vi "Read alarm XML.vi"(0 "map in":T2) -> (7 "map out":T1, 8 "data":T3, 9 "change?":bool)   [LabVIEW 2016, in "Alarm interface.lvlib"]
uses:
  Alarm interface.lvlib
panel:
  out "报警":T4
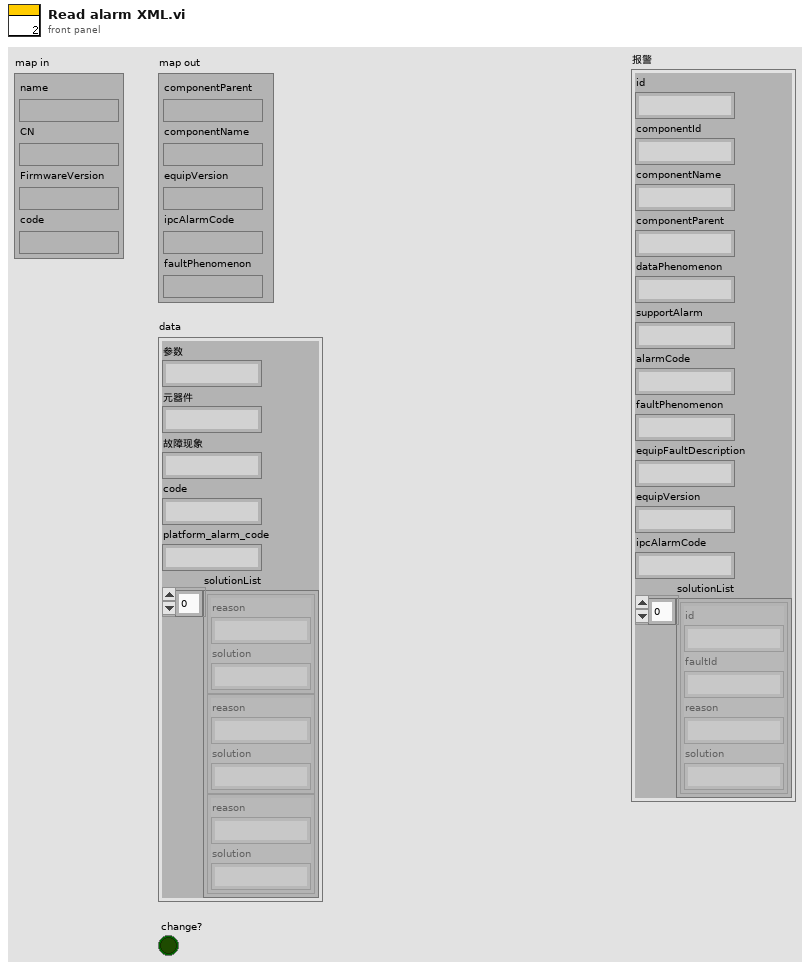
[diagram p1: front panel]
types:
  T1 = typedef "Alarm interface.lvlib/map out.ctl" = cluster{"componentParent":string, "componentName":string, "equipVersion":string, "ipcAlarmCode":string, "faultPhenomenon":string}
  T2 = typedef "Alarm interface.lvlib/map in.ctl" = cluster{"name":string, "CN":string, "FirmwareVersion":string, "code":string}
  T3 = typedef "Alarm interface.lvlib/报警短信语音交互.ctl" = cluster{"参数":string, "元器件":string, "故障现象":string, "code":string, "platform_alarm_code":string, "solutionList":cluster{"reason":string, "solution":string}[]}
  T4 = cluster{"id":string, "componentId":string, "componentName":string, "componentParent":string, "dataPhenomenon":string, "supportAlarm":string, "alarmCode":string, "faultPhenomenon":string, "equipFaultDescription":string, "equipVersion":string, "ipcAlarmCode":string, "solutionList":cluster{"id":string, "faultId":string, "reason":string, "solution":string}[]}
  T5 = cluster{"componentParent":string, "componentName":string, "equipVersion":string, "Code":string}
  T6 = cluster{"id":string, "componentId":string, "componentName":string, "componentParent":string, "dataPhenomenon":string, "supportAlarm":string, "alarmCode":string, "faultPhenomenon":string, "equipFaultDescription":string, "equipVersion":string, "ipcAlarmCode":string, "solutionList":cluster{"id":string, "faultId":string, "reason":string, "solution":string}[]}[]
  T7 = cluster{"id":string, "faultId":string, "reason":string, "solution":string}[]
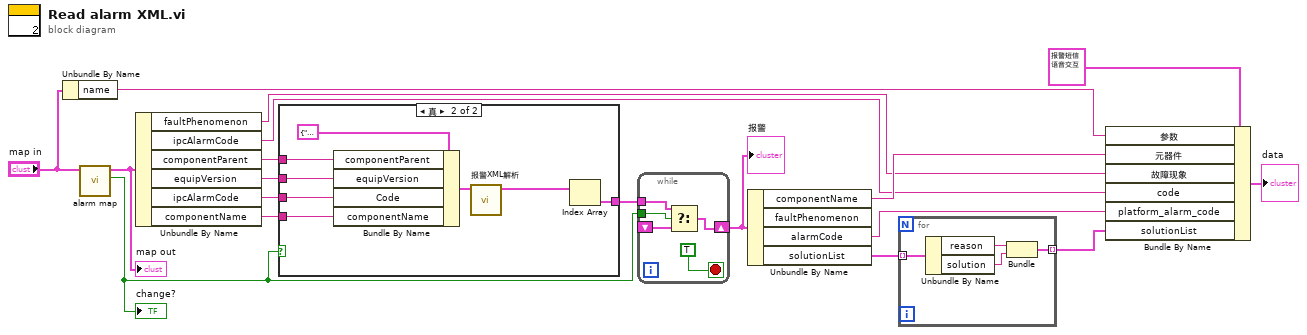
[diagram p0: block diagram]
diagram:
  n1 = Unbundle By Name("map in") -> ("name"=w4:string)
  n2 = call "alarm map.vi"("map in"="map in") -> ("change?"=w6:bool, "map out"=w7:T1)  [unwired: 8 in, 1 out]
  "map out" <- w7
  "change?" <- w6
  n3 = Unbundle By Name(w7) -> ("faultPhenomenon"=w3:string, "ipcAlarmCode"=w2:string, "componentParent"=w17:string, "equipVersion"=w18:string, "ipcAlarmCode"=w8:string, "componentName"=w1:string)
  n4 = case shown="真" w6 {
    tunnel: w17 -> [_ w26]
    tunnel: w18 -> [_ w25]
    tunnel: w8 -> [_ w24]
    tunnel: [_ w22] -> w15
    tunnel: w1 -> [_ w19]
    frame False {
    }
    frame True {
      n5 = Bundle By Name(cluster=T5 {"componentParent"="", "componentName"="", "equipVersion"="", "Code"=""} ("筛选输入"), "componentParent"=w26, "equipVersion"=w25, "Code"=w24, "componentName"=w19) -> (w20:T5)
      n6 = call "报警XML解析.vi"("筛选输入"=w20) -> ("data"=w23:T6)  [unwired: 9 in, 1 out]
      n7 = Index Array(array=w23) -> (element=w22:T4)  [unwired: 1 in]
    }
  }
  n8 = while {
    tunnel: w15 -> [w30]
    shift-right: [w28] -> w14
    shift-left: _ -> [w29]
    tunnel: w6 -> [w31]
    stop <- TRUE stop-if-true
    n9 = Select(t=w30, s=w31, f=w29) -> (s? t:f=w28:T4)
  }
  "报警" <- w14
  n10 = Unbundle By Name(w14) -> ("componentName"=w13:string, "alarmCode"=w12:string, "solutionList"=w11:T7)  [unwired: 1 out]
  n11 = for {
    tunnel: w11 -> [w35] mode=indexing
    tunnel: [w32] -> w9 mode=indexing
    n12 = Unbundle By Name(w35) -> ("reason"=w34:string, "solution"=w33:string)
    n13 = Bundle("reason"=w34, "solution"=w33) -> (w32:cluster{"reason":string, "solution":string})  [unwired: 1 in]
  }
  n14 = Bundle By Name(cluster=T3 {"参数"="", "元器件"="", "故障现象"="", "code"="", "platform_alarm_code"="", "solutionList"=[{"reason"="1、缺标液，", "solution"="1、检查标液口（标液是否用完，及附属管路气密性等），检查管路气密性"}, {"reason"="2、液位传感器异常", "solution"="2、更换液位传感器"}, {"reason"="3、蠕动泵故障或泵管老化导致无法正常抽液", "solution"="3、更换蠕动泵管或更换蠕动泵"}]} ("data"), "参数"=w4, "元器件"=w13, "故障现象"=w3, "code"=w2, "platform_alarm_code"=w12, "solutionList"=w9) -> (→"data":T3)
